vi "Init Double Pneumatics with CVS File.vi"(1 "error in":errorcluster, 2 "Reverse Pnumatic ID":string, 3 "Forward Pnumatic ID":string, 4 "Robot ID":string) -> (0 "error out":errorcluster)   [LabVIEW 2017]
uses:
  <vilib>/Rock Robotics/WPI/SafetyOutput/WPI_SafetyOutputConfigMenu.ctl
  <vilib>/Rock Robotics/WPI/Solenoid/WPI_SolenoidOpenDouble.vi
panel:
  out "Forward Pneumatic Channel":i32
  out "Reverse Pneumatic Channel":i32
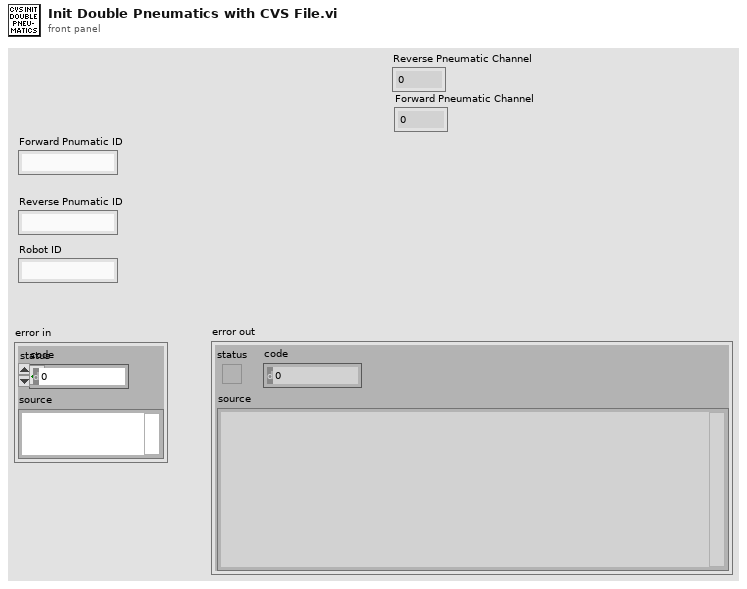
[diagram p1: front panel]
types:
  T1 = typedef "WPI_SafetyOutputConfigMenu.ctl" = enum16{"Enable", "Disable"}
  T2 = typedef "WPI_SolenoidDevRef.ctl" = cluster{"DevStatus":errorcluster, "Pneumatics Control Module":u8, "Forward Solenoid Channel":T3, "Reverse Solenoid Channel":T3}
  T3 = typedef "WPI_SolenoidChannel.ctl" = enum8{"Solenoid 0", "Solenoid 1", "Solenoid 2", "Solenoid 3", "Solenoid 4", "Solenoid 5", "Solenoid 6", "Solenoid 7", "Invalid"}
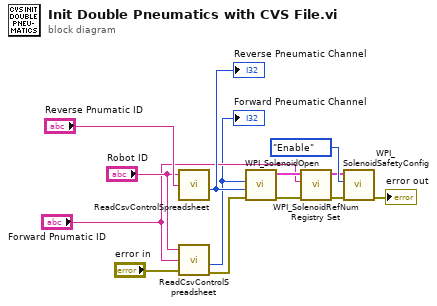
[diagram p0: block diagram]
diagram:
  n1 = call "ReadCsvControlSpreadsheet.vi"("Robot ID"="Robot ID", "Motor ID"="Reverse Pnumatic ID") -> ("Pneumatic Channel"=w4:i32)  [unwired: 1 in, 3 out]
  "Reverse Pneumatic Channel" <- w4
  n2 = call "ReadCsvControlSpreadsheet.vi"("Robot ID"="Robot ID", "Motor ID"="Forward Pnumatic ID", "error in"="error in") -> ("Pneumatic Channel"=w1:i32, "error out"=w7:errorcluster)  [unwired: 2 out]
  "Forward Pneumatic Channel" <- w1
  n3 = call-poly <vilib>:"WPI_SolenoidOpen.vi"("error in (no error)"=w7, "Reverse Solenoid Channel"=w4, "Forward Solenoid Channel"=w1) -> ("error out"=w9:errorcluster, "SolenoidDevRef"=w3:T2)  [unwired: 7 in]
  n4 = call <vilib>:"WPI_SolenoidRefNum Registry Set.vi"("error in (no error)"=w9, "refnum name"="Forward Pnumatic ID", "SolenoidDevRef"=w3) -> ("error out"=w10:errorcluster, "SolenoidDevRef"=w12:T2)  [unwired: 7 in]
  n5 = call <vilib>:"WPI_SolenoidSafetyConfig.vi"("error in (no error)"=w10, "mode"=WPI_SafetyOutputConfigMenu."Enable", "SolenoidDevRef"=w12) -> ("error out"=→"error out":errorcluster)  [unwired: 7 in, 1 out]
